vi "Reports.vi"(0 "SERIAL NUMBER":string, 2 "Result":bool[](array[boolean]), 3 "error in":errorcluster) -> (9 "error out":errorcluster)   [LabVIEW 2019]
uses:
  <vilib>/Utility/file.llb/Write Delimited Spreadsheet (string).vi
panel:
  out "standard error":string
  out "standard output":string
  in  "Header Name":string[](array[string])=["", "", ""]
  in  "JR ENGINEER":string
  in  "RESULT":T1
  in  "S.NO":string
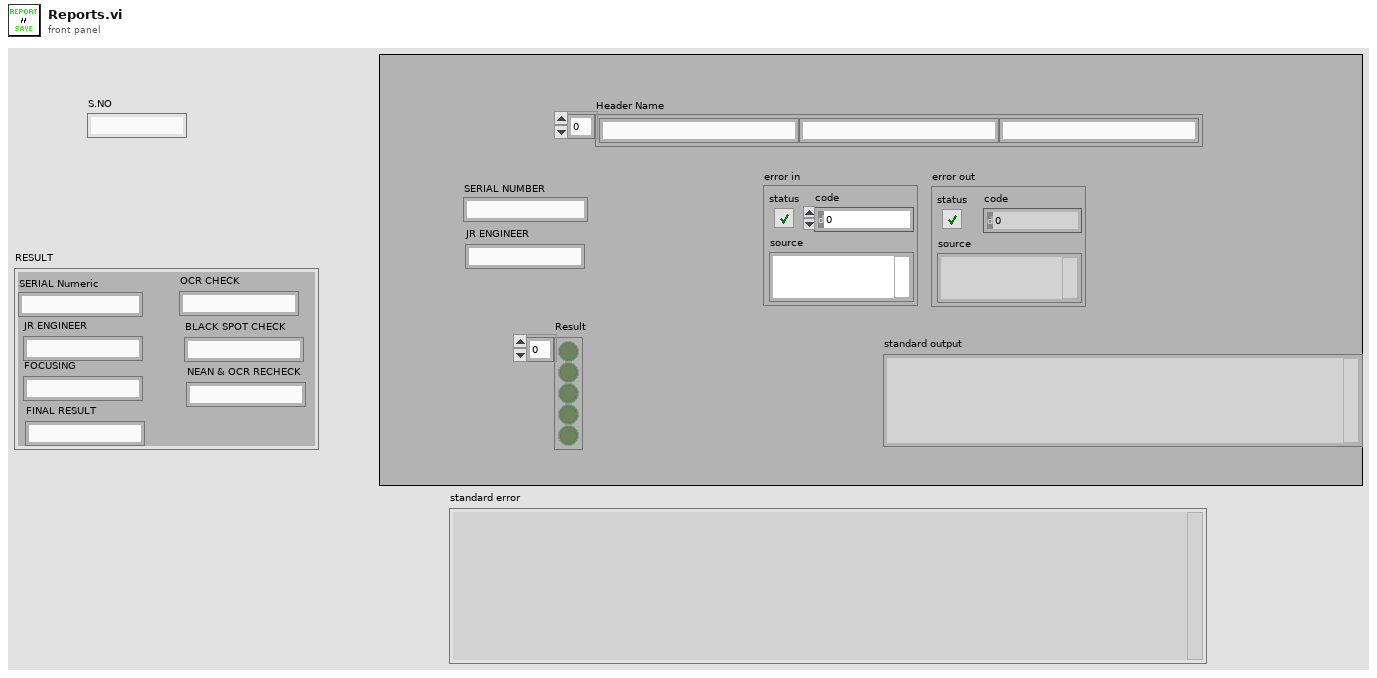
[diagram p1: front panel]
types:
  T1 = cluster{"SERIAL Numeric":string, "JR ENGINEER":string, "FOCUSING":string, "OCR CHECK":string, "BLACK SPOT CHECK":string, "NEAN & OCR RECHECK":string, "FINAL RESULT":string}
  T2 = cluster{"User Login":string, "Password":string, "Default User Type":u16}
  T3 = typedef "IMAQ Image.ctl" = refnum<image>
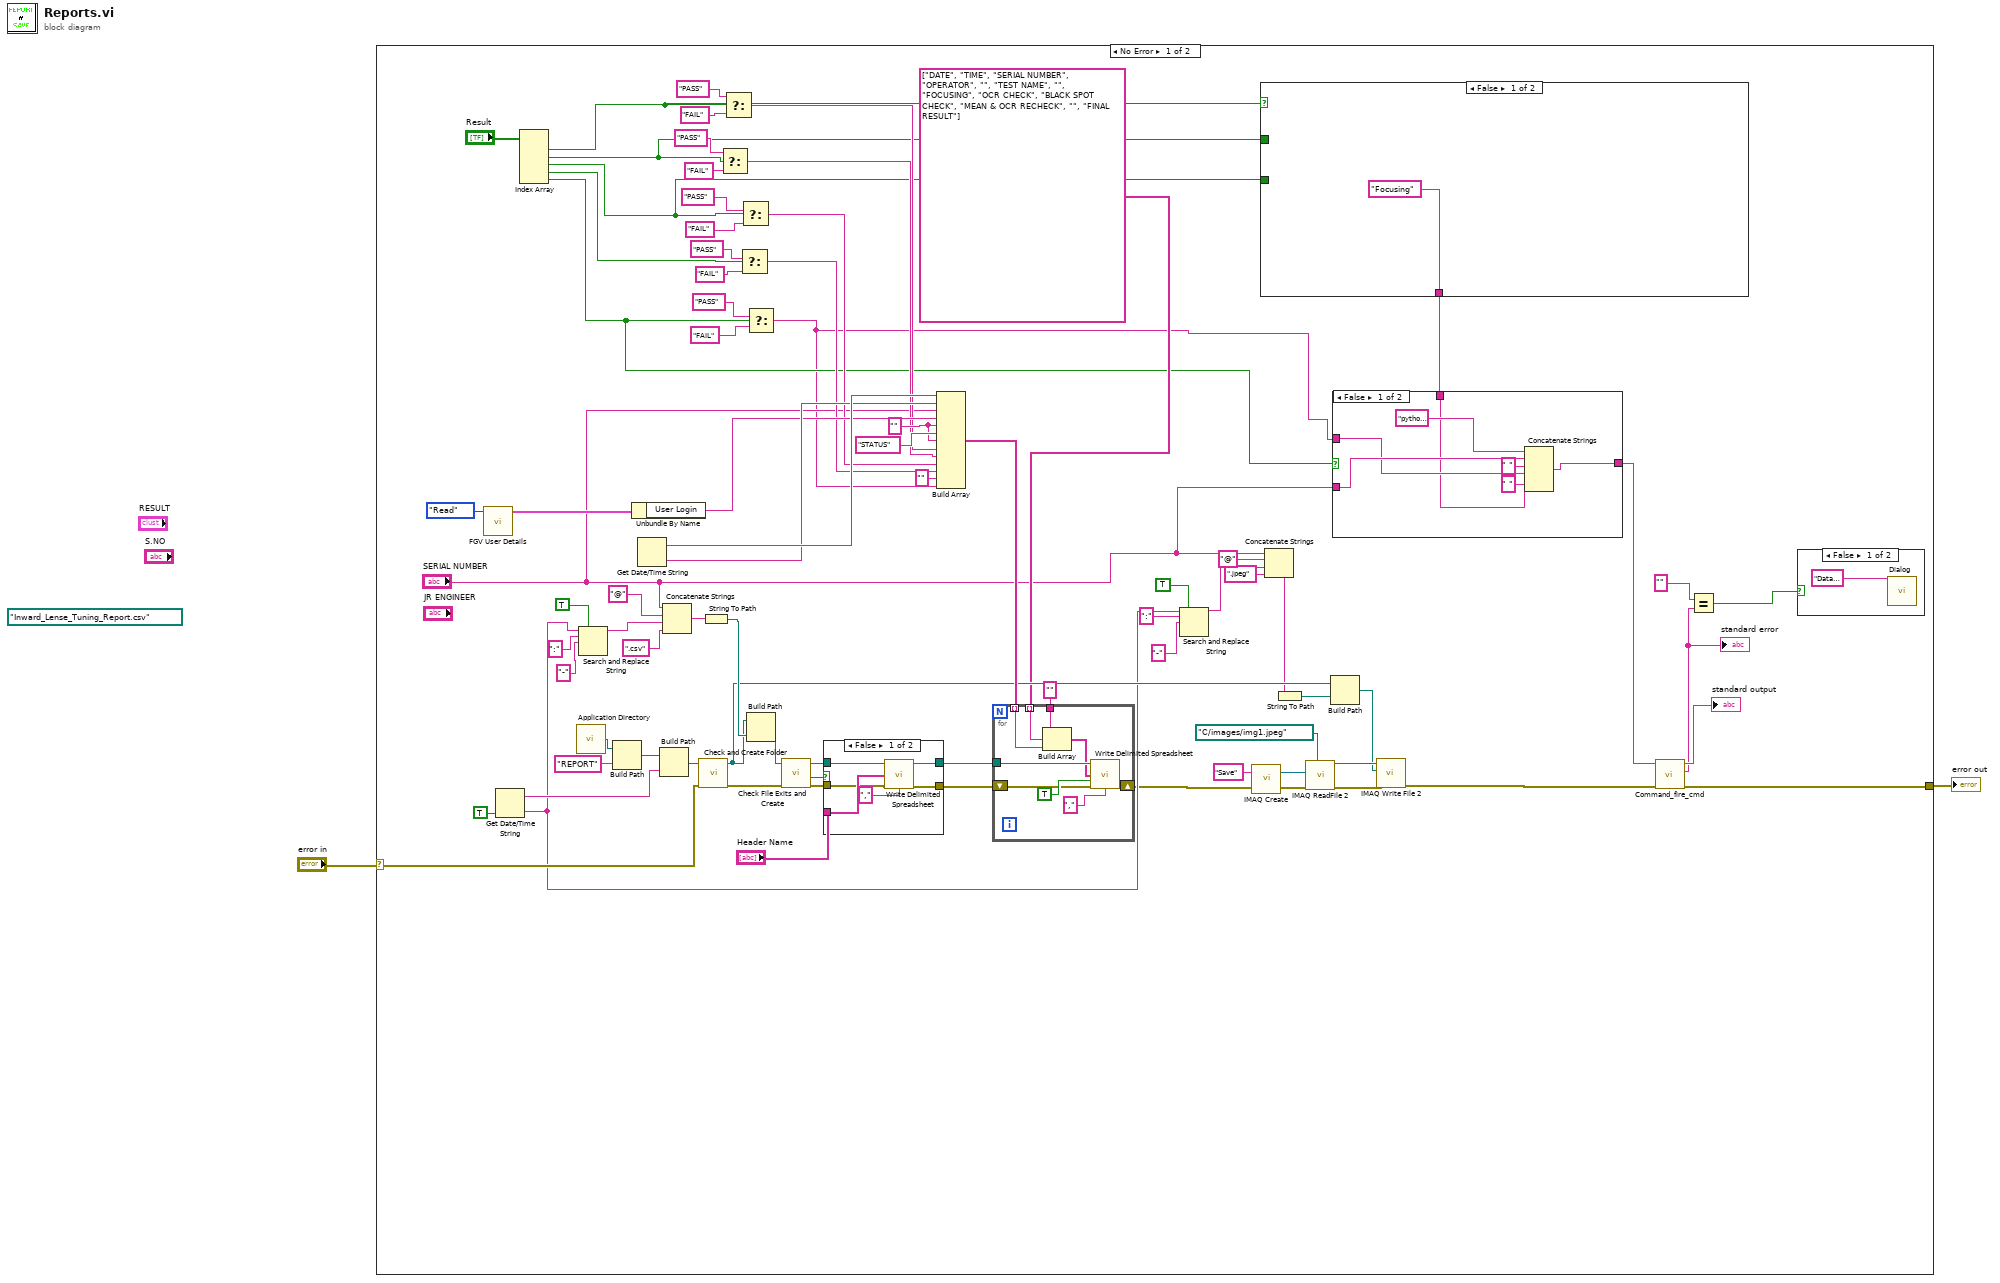
[diagram p0: block diagram]
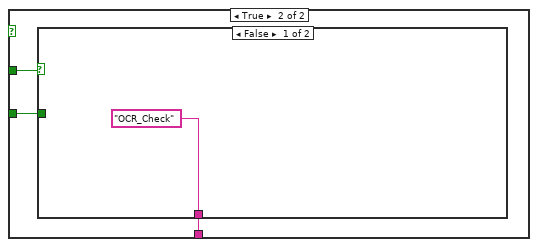
[diagram p3: hidden frame]
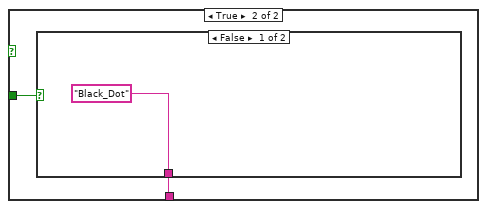
[diagram p4: hidden frame]
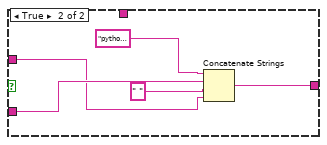
[diagram p6: hidden frame]
diagram:
  (unwired) path "Inward_Lense_Tuning_Report.csv" ("file path (dialog if empty)")
  n1 = case shown="No Error" "error in" {
    selector: "error in" -> [w46 w123]
    tunnel: [w16 w123] -> w2
    frame No Error {
      w25 = "" ("element")
      n2 = call "FGV User Details.vi"("Action"=enum16{"Initialize", "Read", "Write"}."Read") -> ("User Details out"=w48:T2)  [unwired: 9 in, 1 out]
      n3 = Get Date/Time String(want seconds? (F)=TRUE) -> (date string=w73:string, time string=w35:string)  [unwired: 2 in]
      n4 = Index Array(array="Result") -> (element #1=w13:bool, element #2=w12:bool, element #3=w11:bool, element #4=w10:bool, element #5=w15:bool)  [unwired: 5 in]
      n5 = call <vilib>:"Application Directory.vi"() -> ("Application Directory"=w76:path)
      n6 = Search and Replace String(replace all?=TRUE ("replace all? (F)"), input string=w35, search string=":", replace string="-" ("replace string (\"\")")) -> (result string=w63:string)  [unwired: 4 in, 3 out]
      n7 = Build Path(base path=w76, name or relative path="REPORT") -> (appended path=w75:path)
      n8 = Unbundle By Name(w48) -> ("User Login"=w47:string)
      n9 = Get Date/Time String() -> (date string=w71:string, time string=w70:string)  [unwired: 3 in]
      n10 = Build Path(base path=w75, name or relative path=w73) -> (appended path=w74:path)
      n11 = Concatenate Strings("SERIAL NUMBER", "@" ("string"), w63, ".csv" ("string")) -> (w67:string)
      n12 = call "Check and Create Folder.vi"("error in (no error)"=w46, "Path In"=w74) -> ("error out"=w79:errorcluster, "Path Out"=w39:path)  [unwired: 7 in, 1 out]
      n13 = String To Path(string=w67) -> (path=w66:path)
      n14 = Select(t="PASS", s=w12, f="FAIL") -> (s? t:f=w23:string)
      n15 = Select(t="PASS", s=w13, f="FAIL") -> (s? t:f=w24:string)
      n16 = Select(t="PASS", s=w10, f="FAIL") -> (s? t:f=w21:string)
      n17 = Select(t="PASS", s=w11, f="FAIL") -> (s? t:f=w22:string)
      n18 = Select(t="PASS", s=w15, f="FAIL") -> (s? t:f=w6:string)
      n19 = Build Path(base path=w39, name or relative path=w66) -> (appended path=w80:path)
      n20 = call "Check File Exits and Create.vi"("error in"=w79, "Path In"=w80) -> ("error out"=w72:errorcluster, "file exists?"=w78:bool, "Path Out"=w77:path)  [unwired: 6 in, 1 out]
      n21 = case shown="False" w78 {
        tunnel: "Header Name" -> [w119 _]
        tunnel: [w118 w122] -> w84
        tunnel: [w117 w121] -> w82
        tunnel: w77 -> [w116 w122]
        tunnel: w72 -> [w115 w121]
        frame False {
          n22 = call-poly <vilib>:"Write Delimited Spreadsheet.vi"("file path (dialog if empty)"=w116, "1D data"=w119, "error in (no error)"=w115, "delimiter (\\t)"="," ("delimiter (\\t)")) -> ("new file path (Not A Path if cancelled)"=w118:path, "error out"=w117:errorcluster)  [unwired: 10 in]
        }
        frame True {
        }
      }
      n23 = Build Array(w71, w70, "SERIAL NUMBER", w47, w25, "STATUS" ("element"), w25, w24, w23, w22, w21, "" ("element"), w6) -> (w83:string[])
      n24 = for {
        tunnel: w84 -> [w114]
        tunnel: w83 -> [w108] mode=indexing
        shift-right: [w110] -> w28
        shift-left: w82 -> [w111]
        tunnel: string[] ["DATE", "TIME", "SERIAL NUMBER", "OPERATOR", "", "TEST NAME", "", "FOCUSING", "OCR CHECK", "BLACK SPOT CHECK", "MEAN & OCR RECHECK", "", "FINAL RESULT"] -> [w109] mode=indexing
        tunnel: "" ("element") -> [w107]
        n25 = Build Array(w107, w109, w108) -> (w106:string[])
        n26 = call-poly <vilib>:"Write Delimited Spreadsheet.vi"("file path (dialog if empty)"=w114, "1D data"=w106, "append to file? (new file:F)"=TRUE, "error in (no error)"=w111, "delimiter (\\t)"="," ("delimiter (\\t)")) -> ("error out"=w110:errorcluster)  [unwired: 9 in, 1 out]
      }
      n27 = Search and Replace String(replace all?=TRUE ("replace all? (F)"), input string=w35, search string=":", replace string="-" ("replace string (\"\")")) -> (result string=w34:string)  [unwired: 4 in, 3 out]
      n28 = call "IMAQ Create"("Image Name"="Save", "error in (no error)"=w28) -> ("New Image"=w45:T3, "error out"=w43:errorcluster)  [unwired: 3 in]
      n29 = case shown="False" w13 {
        tunnel: w12 -> [_ w89]
        tunnel: w11 -> [_ w88]
        tunnel: ["Focusing" w87] -> w8
        frame False {
        }
        frame True {
          n30 = case shown="False" w89 {
            tunnel: w88 -> [_ w92]
            tunnel: ["OCR_Check" w91] -> w87
            frame False {
            }
            frame True {
              n31 = case shown="False" w92 {
                tunnel: ["Black_Dot" _] -> w91
                frame False {
                }
                frame True {
                }
              }
            }
          }
        }
      }
      n32 = Concatenate Strings("SERIAL NUMBER", "@" ("string"), w34, ".jpeg" ("string")) -> (w31:string)
      n33 = String To Path(string=w31) -> (path=w30:path)
      n34 = call "IMAQ ReadFile 2"("File Path"=path "C:/images/img1.jpeg", "error in (no error)"=w43, "Image"=w45) -> ("error out"=w41:errorcluster, "Image Out"=w42:T3)  [unwired: 4 in, 3 out]
      n35 = Build Path(base path=w39, name or relative path=w30) -> (appended path=w29:path)
      n36 = case shown="False" w15 {
        tunnel: [w100 w105] -> w9
        tunnel: w6 -> [w96 w102]
        tunnel: "SERIAL NUMBER" -> [w98 w103]
        tunnel: w8 -> [w94 _]
        frame False {
          n37 = Concatenate Strings("python C:\\\\Users\\\\vvdn\\\\Downloads\\\\check_upd_db.py ", w98, " " ("string"), w96, " " ("string"), w94) -> (w100:string)
        }
        frame True {
          n38 = Concatenate Strings("python C:\\\\Users\\\\vvdn\\\\Downloads\\\\check_upd_db.py ", w103, " ", w102) -> (w105:string)
        }
      }
      n39 = call-poly "IMAQ Write File 2"("error in (no error)"=w41, "File Path"=w29, "Image"=w42) -> ("error out"=w17:errorcluster)  [unwired: 7 in, 1 out]
      n40 = call "Command_fire_cmd.vi"("error in"=w17, "command line"=w9) -> ("error out"=w16:errorcluster, "standard error"=w4:string, "standard output"=→"standard output":string)  [unwired: 5 in]
      "standard error" <- w4
      n41 = Equal?(x="" ("standard error"), y=w4) -> (x = y?=w3:bool)
      n42 = case shown="False" w3 {
        frame False {
          n43 = call "Dialog.vi"("Status"="Database Connection Error ") -> ()  [unwired: 10 in, 1 out]
        }
        frame True {
        }
      }
    }
    frame Error {
    }
  }
  "error out" <- w2
